vi "Create Ref.vi"(4 "Name":string, 6 "Name Msg":string, 9 "Name Library File Path":path, 10 "Active Project":refnum<vi>) -> (0 "error out":errorcluster, 2 "Ref":T1)   [LabVIEW 2025, in "_Msg Rescript.lvlib" / "_Msg Rescript.lvclass"]
uses:
  _Msg Rescript.lvclass
  Ref.ctl
  Poly VIs.ctl
  <vilib>/Utility/traverseref.llb/TRef TravTarget.ctl
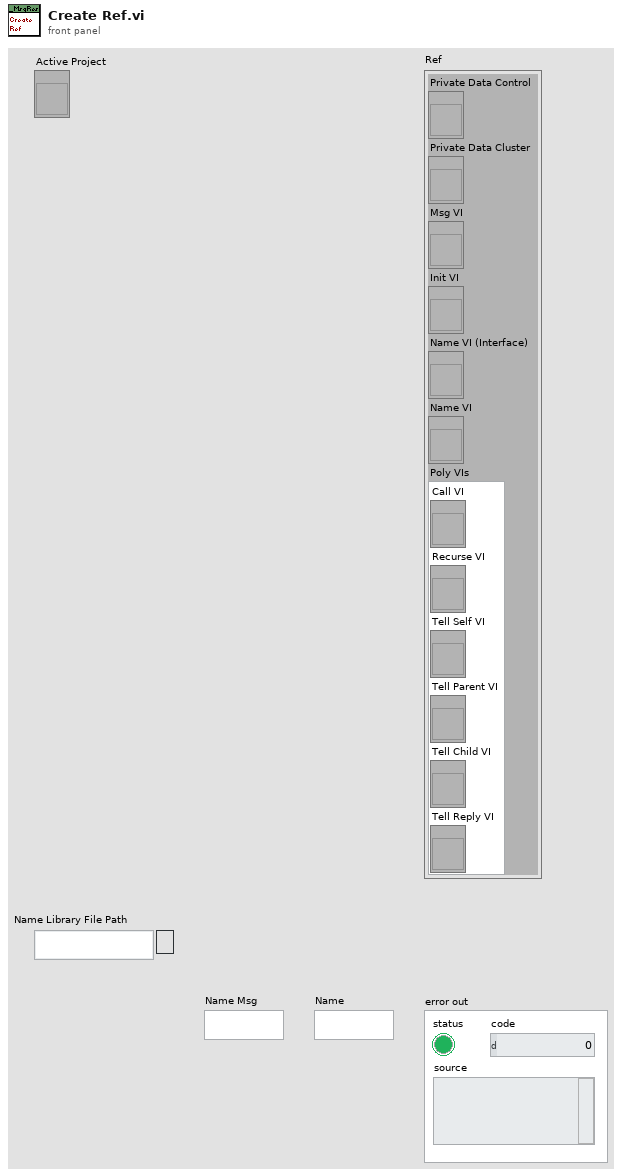
[diagram p1: front panel]
types:
  T1 = typedef "_Msg Rescript.lvlib/_Msg Rescript.lvclass/Ref.ctl" = cluster{"Private Data Control":refnum<vi>, "Private Data Cluster":refnum<vi>, "Msg VI":refnum<vi>, "Init VI":refnum<vi>, "Name VI (Interface)":refnum<vi>, "Name VI":refnum<vi>, "Poly VIs":T2}
  T2 = typedef "_Msg Rescript.lvlib/_Msg Rescript.lvclass/Poly VIs.ctl" = cluster{"Call VI":refnum<vi>, "Recurse VI":refnum<vi>, "Tell Self VI":refnum<vi>, "Tell Parent VI":refnum<vi>, "Tell Child VI":refnum<vi>, "Tell Reply VI":refnum<vi>}
  T3 = typedef "TRef TravTarget.ctl" = enum16{"FP", "BD", "Other"}
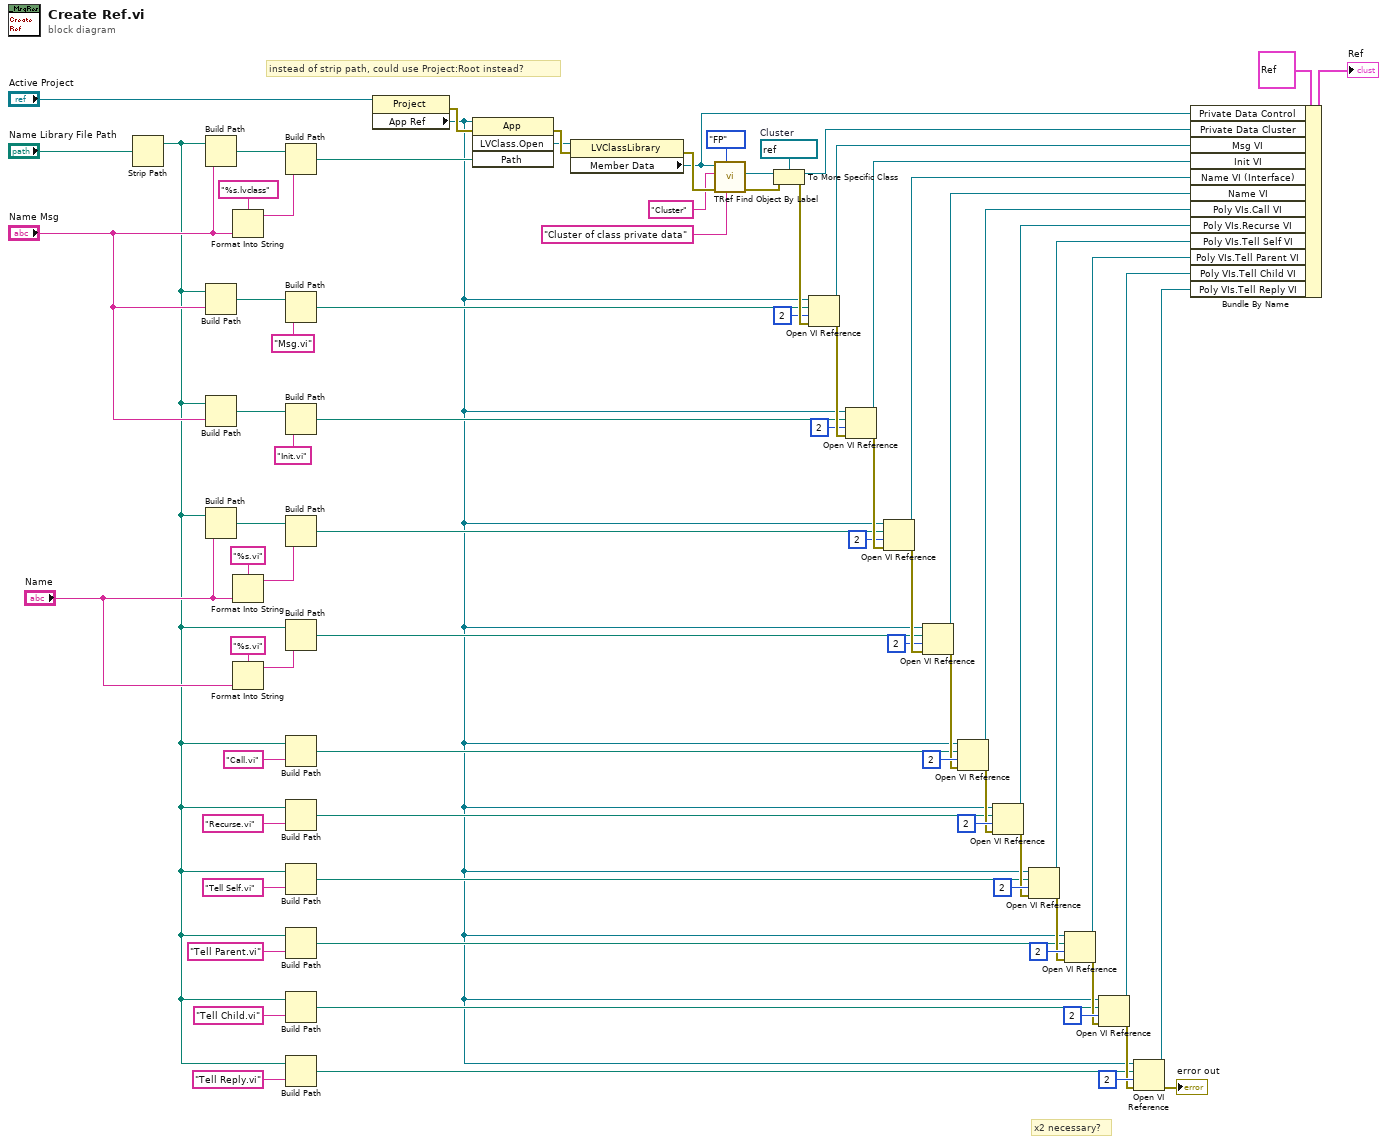
[diagram p0: block diagram]
diagram:
  w72 = refnum<vi> refnum  # Cluster
  # "instead of strip path, could use Project:Root instead?"
  # "x2 necessary?"
  n1 = Strip Path(path="Name Library File Path") -> (stripped path=w4:path)  [unwired: 1 out]
  n2 = Build Path(base path=w4, name or relative path="Name Msg") -> (appended path=w66:path)
  n3 = Build Path(base path=w4, name or relative path="Name Msg") -> (appended path=w59:path)
  n4 = Build Path(base path=w4, name or relative path="Name Msg") -> (appended path=w58:path)
  n5 = Build Path(base path=w4, name or relative path="Name") -> (appended path=w62:path)
  n6 = Format Into String(format string="%s.lvclass", "Name Msg") -> (resulting string=w64:string)  [unwired: 2 in, 1 out]
  n7 = Format Into String(format string="%s.vi", "Name") -> (resulting string=w61:string)  [unwired: 2 in, 1 out]
  n8 = Format Into String(format string="%s.vi", "Name") -> (resulting string=w52:string)  [unwired: 2 in, 1 out]
  n9 = Build Path(base path=w66, name or relative path=w64) -> (appended path=w65:path)
  n10 = Build Path(base path=w59, name or relative path="Msg.vi" ("format string")) -> (appended path=w55:path)
  n11 = Build Path(base path=w58, name or relative path="Init.vi" ("format string")) -> (appended path=w54:path)
  n12 = Build Path(base path=w62, name or relative path=w61) -> (appended path=w50:path)
  n13 = Build Path(base path=w4, name or relative path=w52) -> (appended path=w51:path)
  n14 = Build Path(base path=w4, name or relative path="Call.vi" ("format string")) -> (appended path=w13:path)
  n15 = Build Path(base path=w4, name or relative path="Recurse.vi" ("format string")) -> (appended path=w12:path)
  n16 = Build Path(base path=w4, name or relative path="Tell Self.vi" ("format string")) -> (appended path=w11:path)
  n17 = Build Path(base path=w4, name or relative path="Tell Parent.vi" ("format string")) -> (appended path=w10:path)
  n18 = Build Path(base path=w4, name or relative path="Tell Child.vi" ("format string")) -> (appended path=w9:path)
  n19 = Build Path(base path=w4, name or relative path="Tell Reply.vi" ("format string")) -> (appended path=w3:path)
  n20 = property class="Project"(reference="Active Project") -> (error out=w76:errorcluster, "App Ref"=w1:refnum<vi>)  [unwired: 1 in, 1 out]
  n21 = invoke class="App" method="LVClass.Open"(reference=w1, error in=w76, "Path"=w65) -> (error out=w74:errorcluster, "LVClass.Open"=w67:refnum<vi>)  [unwired: 1 in, 2 out]
  n22 = property class="LVClassLibrary"(reference=w67, error in=w74) -> (error out=w80:errorcluster, "Member Data"=w34:refnum<vi>)  [unwired: 1 out]
  n23 = call <vilib>:"TRef Find Object By Label.vi"("Label"="Cluster of class private data" ("Class Name"), "Traverse Target"=TRef_TravTarget."FP", "error in (no error)"=w80, "Class Name"="Cluster", "VI Ref"=w34) -> ("error out"=w73:errorcluster, "Found Obj Ref"=w71:refnum<vi>)  [unwired: 3 in, 2 out]
  n24 = To More Specific Class(target class=w72, reference=w71, error in=w73) -> (specific class reference=w39:refnum<vi>, error out=w75:errorcluster)
  n25 = Open VI Reference(application reference (local)=w1, vi path=w55, options=2, error in (no error)=w75) -> (vi reference=w40:refnum<vi>, error out=w79:errorcluster)  [unwired: 2 in]
  n26 = Open VI Reference(application reference (local)=w1, vi path=w54, options=2, error in (no error)=w79) -> (vi reference=w41:refnum<vi>, error out=w78:errorcluster)  [unwired: 2 in]
  n27 = Open VI Reference(application reference (local)=w1, vi path=w50, options=2, error in (no error)=w78) -> (vi reference=w42:refnum<vi>, error out=w77:errorcluster)  [unwired: 2 in]
  n28 = Open VI Reference(application reference (local)=w1, vi path=w51, options=2, error in (no error)=w77) -> (vi reference=w43:refnum<vi>, error out=w23:errorcluster)  [unwired: 2 in]
  n29 = Open VI Reference(application reference (local)=w1, vi path=w13, options=2, error in (no error)=w23) -> (vi reference=w28:refnum<vi>, error out=w22:errorcluster)  [unwired: 2 in]
  n30 = Open VI Reference(application reference (local)=w1, vi path=w12, options=2, error in (no error)=w22) -> (vi reference=w27:refnum<vi>, error out=w21:errorcluster)  [unwired: 2 in]
  n31 = Open VI Reference(application reference (local)=w1, vi path=w11, options=2, error in (no error)=w21) -> (vi reference=w26:refnum<vi>, error out=w20:errorcluster)  [unwired: 2 in]
  n32 = Open VI Reference(application reference (local)=w1, vi path=w10, options=2, error in (no error)=w20) -> (vi reference=w25:refnum<vi>, error out=w19:errorcluster)  [unwired: 2 in]
  n33 = Open VI Reference(application reference (local)=w1, vi path=w9, options=2, error in (no error)=w19) -> (vi reference=w24:refnum<vi>, error out=w6:errorcluster)  [unwired: 2 in]
  n34 = Open VI Reference(application reference (local)=w1, vi path=w3, options=2, error in (no error)=w6) -> (vi reference=w2:refnum<vi>, error out=→"error out":errorcluster)  [unwired: 2 in]
  n35 = Bundle By Name(cluster=T1 {"Private Data Control"=refnum, "Private Data Cluster"=refnum, "Msg VI"=refnum, "Init VI"=refnum, "Name VI (Interface)"=refnum, "Name VI"=refnum, "Poly VIs"={"Call VI"=refnum, "Recurse VI"=refnum, "Tell Self VI"=refnum, "Tell Parent VI"=refnum, "Tell Child VI"=refnum, "Tell Reply VI"=refnum}} ("Ref"), "Private Data Control"=w34, "Private Data Cluster"=w39, "Msg VI"=w40, "Init VI"=w41, "Name VI (Interface)"=w42, "Name VI"=w43, "Poly VIs.Call VI"=w28, "Poly VIs.Recurse VI"=w27, "Poly VIs.Tell Self VI"=w26, "Poly VIs.Tell Parent VI"=w25, "Poly VIs.Tell Child VI"=w24, "Poly VIs.Tell Reply VI"=w2) -> (→"Ref":T1)
